vi "Nitro_Pressure.vi"() -> ()   [LabVIEW 2018]
panel:
  in  "End Loop":bool
  in  "Temp":dbl
  out "?":dbl
  out "Nitro Pressure":dbl(knob) scale=0.0..7500.0
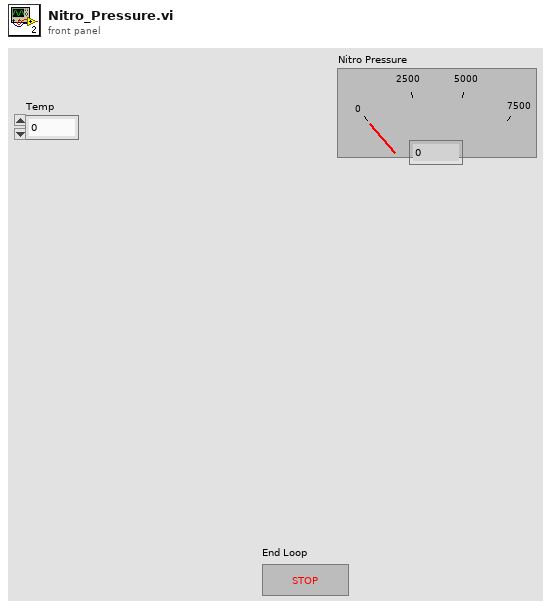
[diagram p1: front panel]
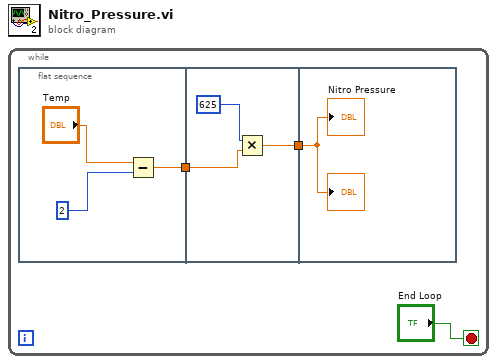
[diagram p0: block diagram]
diagram:
  n1 = while {
    stop <- "End Loop" stop-if-true
    n2 = flat-sequence {
      tunnel: [w4] -> w3
      tunnel: w3 -> [w8]
      tunnel: [w7] -> w2
      tunnel: w2 -> [w10]
      frame #0 {
        n3 = Subtract(x="Temp", y=2) -> (x-y=w4:dbl)
      }
      frame #1 {
        n4 = Multiply(x=625, y=w8) -> (x*y=w7:dbl)
      }
      frame #2 {
        "Nitro Pressure" <- w10
        "?" <- w10
      }
    }
  }
